vi "Scott -- strain -- read multiple voltages SRS.vi"(8 "error IN":errorcluster, 11 "Lockin Settings IN":cluster{"Offset":bool, "GPIB Address":i16}[](array[cluster])) -> (0 "error OUT":errorcluster, 2 "voltages":dbl[](array[numeric]))   [LabVIEW 2014]
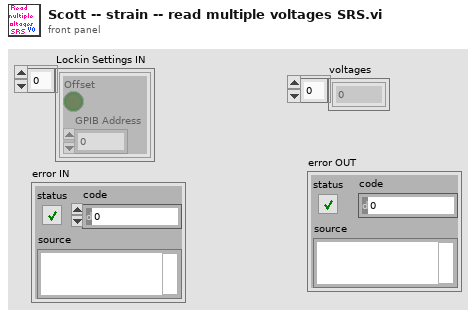
[diagram p1: front panel]
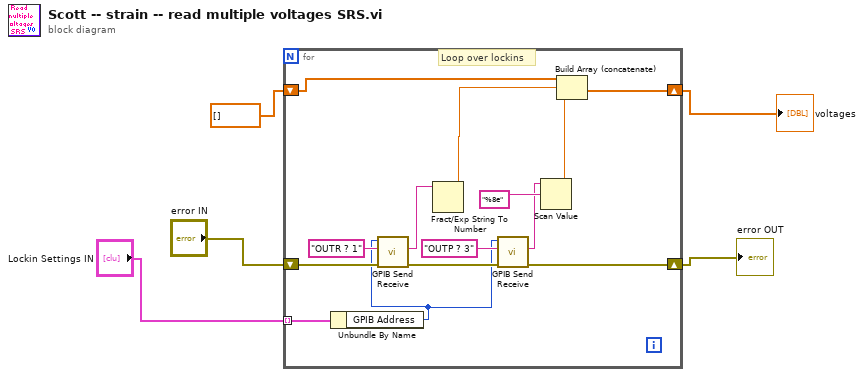
[diagram p0: block diagram]
diagram:
  n1 = for {
    shift-right: [w10] -> w5
    shift-left: dbl[] [] -> [w9]
    shift-right: [w13] -> w1
    shift-left: "error IN" -> [w8]
    tunnel: "Lockin Settings IN" -> [w7] mode=indexing
    # "Loop over lockins"
    n2 = Unbundle By Name(w7) -> ("GPIB Address"=w6:i16)
    n3 = call "GPIB Send Receive.vi"("error in (no error)"=w8, "data string in"="OUTR ? 1", "GPIB Adress"=w6) -> ("error out"=w19:errorcluster, "data string out"=w16:string)  [unwired: 6 in, 1 out]
    n4 = Fract/Exp String To Number(string=w16) -> (number=w11:dbl)  [unwired: 3 in, 1 out]
    n5 = call "GPIB Send Receive.vi"("error in (no error)"=w19, "data string in"="OUTP ? 3", "GPIB Adress"=w6) -> ("error out"=w13:errorcluster, "data string out"=w14:string)  [unwired: 6 in, 1 out]
    n6 = Scan Value(string=w14, format string="%8e") -> (value=w12:dbl)  [unwired: 1 in, 1 out]
    n7 = Build Array (concatenate)(w9, w11, w12) -> (w10:dbl[])
  }
  "voltages" <- w5
  "error OUT" <- w1
